vi "Retrieve Response_core.vi"(8 "error in (no error)":errorcluster, 11 "HttpResponseMessage in":refnum<class "HttpResponseMessage.lvclass">) -> (0 "error out":errorcluster, 1 "Status":i32(ring) items=["Created", "WaitingForActivation", "WaitingToRun", "Running", "WaitingForChildrenToComplete", "RanToCompletion", "Canceled", "Faulted"], 2 "HttpResponseMessage":refnum<k24>, 3 "HttpResponseMessage out":refnum<class "HttpResponseMessage.lvclass">)   [LabVIEW 2024, in "HttpClient_NET.lvlib" / "HttpResponseMessage.lvclass"]
doc: "<b> </b> <b> </b>\nHttpClient_NET\nJustin Young - Viviota\nCopyright (c) 2021\nLicense: BSD"
uses:
  HttpResponseMessage.lvclass
  HttpResponseMessage.lvclass/HttpResponseMessage.ctl
  HttpClient_NET.lvlib
  Types/HttpNet_error_enum.ctl
  System.Net.Http
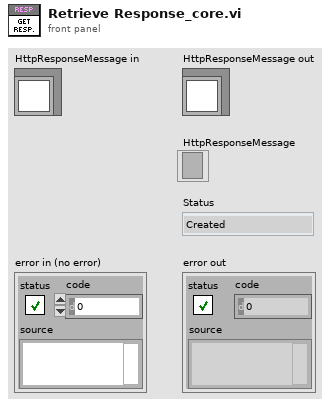
[diagram p1: front panel]
types:
  T1 = typedef "HttpClient_NET.lvlib/HttpNet_error_enum.ctl" = enum16{"REST method is not available", "URL cannot be blank", "Output filepath cannot be empty", "Input filepath cannot be empty", "Internal .NET error %s", "Output filepath cannot be directory", "Download Task no longer exists", "Mutipart Put not supported from REST Client Interface.  Please revert to lower level classes"}
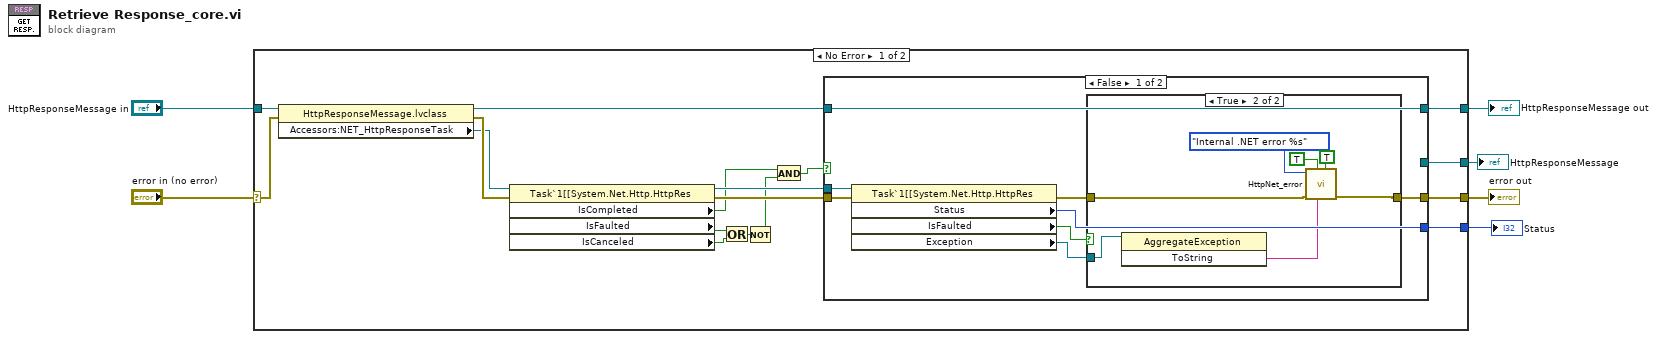
[diagram p0: block diagram]
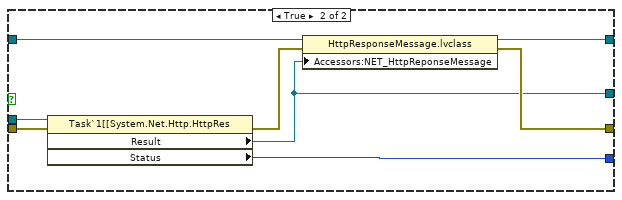
[diagram p3: hidden frame]
diagram:
  n1 = case shown="No Error" "error in (no error)" {
    selector: "error in (no error)" -> [w23 w49]
    tunnel: [w19 w49] -> w5
    tunnel: [w17 w48] -> w3
    tunnel: "HttpResponseMessage in" -> [w21 w48]
    tunnel: [w20 _] -> w2
    tunnel: [w13 _] -> w1
    frame No Error {
      n2 = property class="HttpResponseMessage.lvclass"(reference=w21, error in=w23) -> (reference out=w18:refnum<class "HttpResponseMessage.lvclass">, error out=w22:errorcluster, "Accessors:NET_HttpResponseTask"=w15:refnum<k24>)
      n3 = property class="Task`1[[System.Net.Http.HttpRes"(reference=w15, error in=w22) -> (reference out=w14:refnum<k24>, error out=w16:errorcluster, "IsCompleted"=w12:bool, "IsFaulted"=w10:bool, "IsCanceled"=w9:bool)
      n4 = Or(x=w10, y=w9) -> (x .or. y?=w8:bool)
      n5 = Not(x=w8) -> (.not. x?=w7:bool)
      n6 = And(x=w12, y=w7) -> (x .and. y?=w11:bool)
      n7 = case shown="False" w11 {
        tunnel: [w29 w46] -> w20
        tunnel: [w26 w45] -> w19
        tunnel: w18 -> [w28 w44]
        tunnel: [w28 w43] -> w17
        tunnel: w16 -> [w31 w42]
        tunnel: w14 -> [w30 w41]
        tunnel: [_ w40] -> w13
        frame False {
          n8 = property class="Task`1[[System.Net.Http.HttpRes"(reference=w30, error in=w31) -> (error out=w27:errorcluster, "Status"=w29:i32, "IsFaulted"=w25:bool, "Exception"=w24:refnum<k24>)  [unwired: 1 out]
          n9 = case shown="True" w25 {
            tunnel: [w32 w36] -> w26
            tunnel: w24 -> [_ w39]
            tunnel: w27 -> [w32 w37]
            frame False {
            }
            frame True {
              n10 = invoke class="AggregateException" method="ToString"(reference=w39) -> ("ToString"=w38:string)  [unwired: 2 in, 2 out]
              n11 = call "HttpNet_error.vi"("ShowCallChain [T]"=TRUE, "IncludedString"=w38, "OverrideExistingErrors [T]"=TRUE, "Error In"=w37, "Error"=HttpNet_error_enum."Internal .NET error %s") -> ("Error Out"=w36:errorcluster)  [unwired: 6 in]
            }
          }
        }
        frame True {
          n12 = property class="Task`1[[System.Net.Http.HttpRes"(reference=w41, error in=w42) -> (error out=w47:errorcluster, "Result"=w40:refnum<k24>, "Status"=w46:i32)  [unwired: 1 out]
          n13 = property class="HttpResponseMessage.lvclass"(reference=w44, error in=w47, "Accessors:NET_HttpReponseMessage"=w40) -> (reference out=w43:refnum<class "HttpResponseMessage.lvclass">, error out=w45:errorcluster)
        }
      }
    }
    frame Error {
    }
  }
  "error out" <- w5
  "HttpResponseMessage out" <- w3
  "Status" <- w2
  "HttpResponseMessage" <- w1
